vi "CRYInsert All to Listbox Etc.vi"(7 "sAction":string) -> ()   [LabVIEW 2013]
panel:
  # "Insert All(Curve, Value, Result, Waveform) to Listbox"
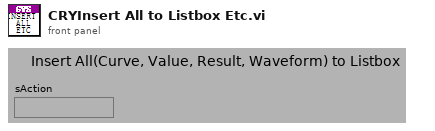
[diagram p1: front panel]
types:
  T1 = typedef "CRYData Cluster.ctl" = cluster{"Name":string, "Curve":cluster{"x":dbl, "y":dbl, "z":dbl}[], "X data":u16, "Y data":u16, "Z data":u16, "X axis":u16, "Y axis":u16, "Z axis":u16, "X unit":string, "Y unit":string, "Z unit":string, "X dB ref":dbl, "Y dB ref":dbl, "Z dB ref":dbl, "single val":bool, "protected":bool, "display X":bool, "display Y":bool, "display Z":bool, "Test Info":string, "Step No.":i32, "Plot Settings":cluster{"Color":u32, "Interpolation":u8, "Point Style":u8, "Line Style":u8, "Point Color":u32, "Line Width":u8, "Bar Plot Style":u8, "Fill To":i16}, "AutoProtect":bool}
  T2 = typedef "CRYWaveform Cluster.ctl" = cluster{"Waveform":cluster{"X0":dbl, "dX":dbl, "Y":sgl[]}, "X data":u16, "Y data":u16, "Y axis":u16, "X unit":string, "Y unit":string, "Y dB ref":dbl, "display Y":bool, "display X":bool, "Overload?":bool, "Test Info":string, "Step No.":i32, "Name":string, "protected":bool, "Sqc history":string[], "Signal Channel ID":i32, "Plot Settings":cluster{"Color":u32, "Interpolation":u8, "Point Style":u8, "Line Style":u8, "Point Color":u32, "Line Width":u8, "Bar Plot Style":u8, "Fill To":i16}, "AutoProtect":bool}
  T3 = typedef "CRYResult Cluster.ctl" = cluster{"Name":string, "Margin":dbl, "unit":string, "Verdict":bool, "Limit":string, "Max/Min":string, "protected":bool, "Step No.":i32, "Test Info":string, "AutoProtect":bool}
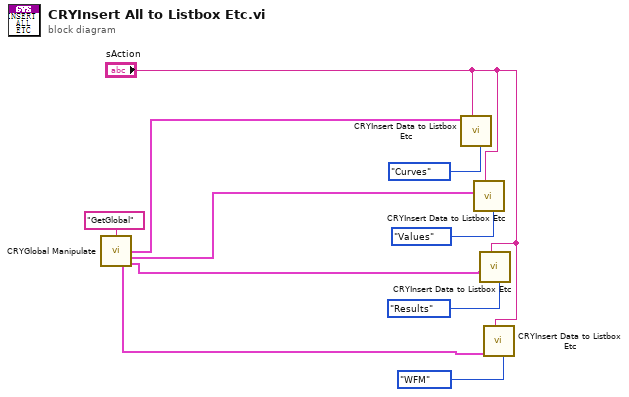
[diagram p0: block diagram]
diagram:
  n1 = call "CRYGlobal Manipulate.vi"("sAction"="GetGlobal") -> ("Curves Out"=w8:T1[], "Values Out"=w7:T1[], "WFM Out"=w3:T2[], "Results Out"=w5:T3[])  [unwired: 8 in, 3 out]
  n2 = call "CRYInsert Data to Listbox Etc.vi"("Type"=enum16{"Curves", "Values", "Results", "WFM"}."Curves", "sAction"="sAction", "Curves"=w8) -> ()  [unwired: 9 in]
  n3 = call "CRYInsert Data to Listbox Etc.vi"("Type"=enum16{"Curves", "Values", "Results", "WFM"}."Values", "sAction"="sAction", "Values"=w7) -> ()  [unwired: 9 in]
  n4 = call "CRYInsert Data to Listbox Etc.vi"("Type"=enum16{"Curves", "Values", "Results", "WFM"}."Results", "sAction"="sAction", "Results"=w5) -> ()  [unwired: 9 in]
  n5 = call "CRYInsert Data to Listbox Etc.vi"("Type"=enum16{"Curves", "Values", "Results", "WFM"}."WFM", "sAction"="sAction", "Waveforms"=w3) -> ()  [unwired: 9 in]
